vi "SET_OUTPUT_POWER.vi"(7 "LabVIEW Web Service Request":refnum<class "Web Request.lvclass">, 9 "OUTPUT":bool, 10 "VBAT":dbl, 11 "DEVICE":string) -> (3 "Response":T1)   [LabVIEW 2015]
uses:
  <vilib>/wsapi/Web Request.lvclass
  Share Data/uPower_kit.ctl
panel:
  # "Use the Web Service Request input terminal to call the VIs on the Web Services palette. Do not remove it from the connector pane unless you don't need access to the palette."
  # "Each additional control wired to the connector pane will be available as an input in the URL. To include an indicator in terminal-mode output (the default setting), it must also be wired to the connector pane."
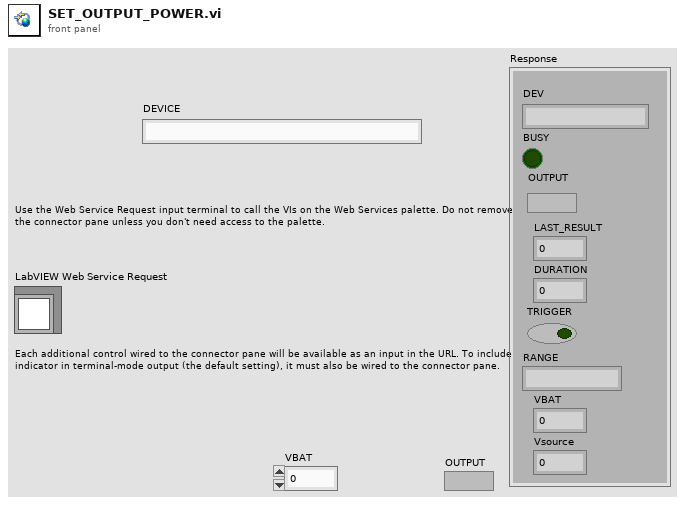
[diagram p1: front panel]
types:
  T1 = typedef "uPower_kit.ctl" = cluster{"DEV":string, "BUSY":bool, "VBAT":dbl, "OUTPUT":bool, "LAST_RESULT":dbl, "DURATION":u16, "TRIGGER":bool, "RANGE":string, "Vsource":dbl}
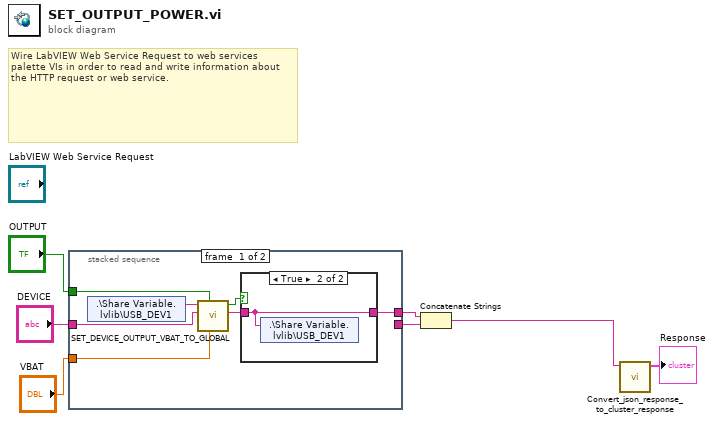
[diagram p0: block diagram]
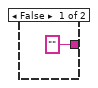
[diagram p2: hidden frame]
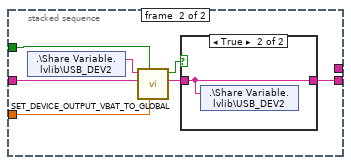
[diagram p3: hidden frame]
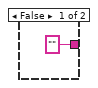
[diagram p4: hidden frame]
diagram:
  # "Wire LabVIEW Web Service Request to web services palette VIs in order to read and write information about the HTTP request or web service."
  n1 = stacked-sequence {
    tunnel: "OUTPUT" -> [w12 w21]
    tunnel: "DEVICE" -> [w11 w20]
    tunnel: [w9 _] -> w5
    tunnel: [_ w18] -> w4
    tunnel: "VBAT" -> [w8 w17]
    frame #0 {
      n2 = shared-variable ".\\Share Variable.lvlib\\USB_DEV1"() -> (w14:string)  [unwired: 1 in, 1 out]
      n3 = call "SET_DEVICE_OUTPUT_VBAT_TO_GLOBAL.vi"("VBAT"=w8, "OUTPUT"=w12, "DEVICE"=w11, "USB_DEV"=w14) -> ("JSON string response TO USB DEV"=w13:string, "Dev?"=w10:bool)  [unwired: 6 in]
      n4 = case shown="True" w10 {
        tunnel: w13 -> [_ w16]
        tunnel: ["" ("JSON string response TO USB DEV") w16] -> w9
        frame False {
        }
        frame True {
          n5 = shared-variable ".\\Share Variable.lvlib\\USB_DEV1"(w16) -> ()  [unwired: 1 in, 1 out]
        }
      }
    }
    frame #1 {
      n6 = shared-variable ".\\Share Variable.lvlib\\USB_DEV2"() -> (w23:string)  [unwired: 1 in, 1 out]
      n7 = call "SET_DEVICE_OUTPUT_VBAT_TO_GLOBAL.vi"("VBAT"=w17, "OUTPUT"=w21, "DEVICE"=w20, "USB_DEV"=w23) -> ("JSON string response TO USB DEV"=w22:string, "Dev?"=w19:bool)  [unwired: 6 in]
      n8 = case shown="True" w19 {
        tunnel: w22 -> [_ w25]
        tunnel: ["" ("JSON string response TO USB DEV") w25] -> w18
        frame False {
        }
        frame True {
          n9 = shared-variable ".\\Share Variable.lvlib\\USB_DEV2"(w25) -> ()  [unwired: 1 in, 1 out]
        }
      }
    }
  }
  n10 = Concatenate Strings(w5, w4) -> (w2:string)
  n11 = call "Convert_json_response_to_cluster_response.vi"("Json_Response_in"=w2) -> ("Response"=→"Response":T1)  [unwired: 10 in]
